vi "TIcks per decisecond to Rotations per second.vi"(11 "Drive Velocities (ticks/ds)":T1) -> (3 "Drive Velocities (rotations/s)":T1)   [LabVIEW 2020]
uses:
  2023 Charged Up Robot Project/Framework/Robot Global Data.vi
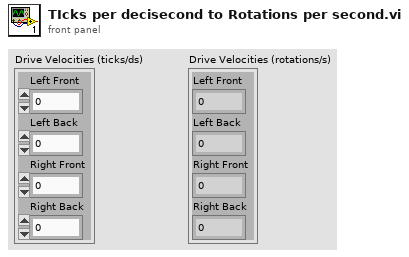
[diagram p1: front panel]
types:
  T1 = cluster{"Left Front":dbl, "Left Back":dbl, "Right Front":dbl, "Right Back":dbl}
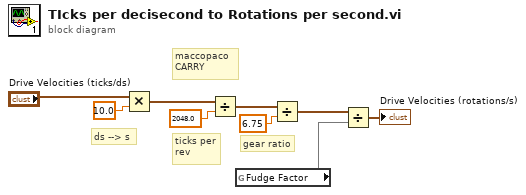
[diagram p0: block diagram]
diagram:
  # "ds --> s"
  # "ticks per\nrev"
  # "gear ratio"
  # "maccopaco\nCARRY"
  n1 = Multiply(x="Drive Velocities (ticks/ds)", y=10.0) -> (x*y=w2:T1)
  n2 = Divide(x=w2, y=2048.0) -> (x/y=w1:T1)
  n3 = global read "Robot Global Data.vi" "Fudge Factor"() -> (w4)
  n4 = Divide(x=w1, y=6.75) -> (x/y=w5:T1)
  n5 = Divide(x=w5, y=w4) -> (x/y=→"Drive Velocities (rotations/s)":T1)
